vi "readFromXML.vi"(8 "error in (no error)":errorcluster, 10 "XML in":string, 11 "Guide in":refnum<class "Guide.lvclass">) -> (0 "error out":errorcluster, 3 "Guide out":refnum<class "Guide.lvclass">)   [LabVIEW 2022 SP3, in "TCSDataDefinitions.lvlib" / "TCSCommand.lvlib" / "GuiderCommands.lvlib" / "Guide.lvclass"]
uses:
  Guide.lvclass
  Enumerations/GuideStateTypes.ctl
  Guide.lvclass/Guide.ctl
  GuiderCommands.lvclass
  <userlib>/Common/XML/XMLParser/XMLParser.lvclass
  TCSCommand.lvlib
panel:
  out "guideStateTypes":T1
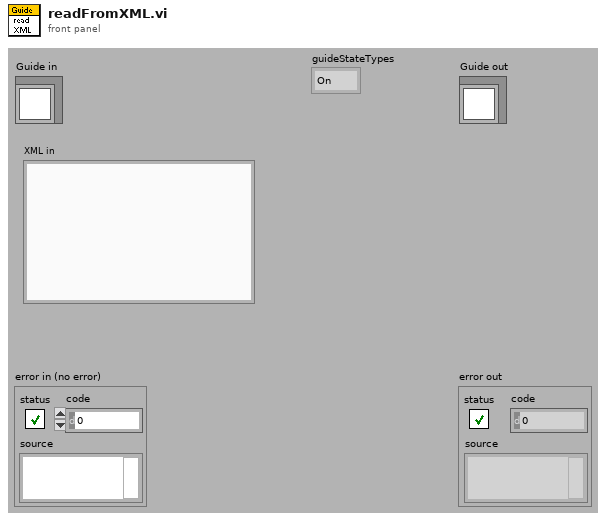
[diagram p1: front panel]
types:
  T1 = typedef "TCSDataDefinitions.lvlib/TCSCommand.lvlib/GuideStateTypes.ctl" = enum16{"On", "Off"}
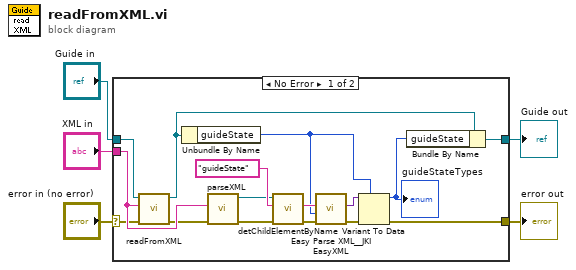
[diagram p0: block diagram]
diagram:
  n1 = case shown="No Error" "error in (no error)" {
    selector: "error in (no error)" -> [w15 w23]
    tunnel: [w9 w23] -> w4
    tunnel: [w19 w22] -> w2
    tunnel: "Guide in" -> [w18 w22]
    tunnel: "XML in" -> [w16 _]
    frame No Error {
      n2 = call-parent "readFromXML.vi"("error in (no error)"=w15, "XMLin"=w16, "GuiderCommands in"=w18) -> ("error out"=w14:errorcluster, "GuiderCommands out"=w17:refnum<class "Guide.lvclass">)  [unwired: 7 out]
      n3 = Unbundle By Name(w17) -> ("guideState"=w7:T1)
      n4 = call <userlib>:"parseXML.vi"("error in (no error)"=w14, "XMLString in"=w16) -> ("error out"=w20:errorcluster, "Element out"=w6:refnum<class "XMLParser.lvclass">)  [unwired: 8 in]
      n5 = call <userlib>:"detChildElementByName.vi"("error in (no error)"=w20, "childName"="guideState" ("ChildName"), "Element in"=w6) -> ("error out"=w10:errorcluster, "childXML"=w11:string)  [unwired: 5 in, 2 out]
      n6 = call <vilib>:"Easy Parse XML__JKI EasyXML.vi"("error in (no error)"=w10, "LabVIEW Data (Type)"=w7, "XML String"=w11) -> ("error out"=w13:errorcluster, "LabVIEW Data"=w12:variant)  [unwired: 7 in]
      n7 = Variant To Data(error in=w13, type=w7, Variant=w12) -> (data=w8:T1, error out=w9:errorcluster)
      "guideStateTypes" <- w8
      n8 = Bundle By Name(cluster=w17, "guideState"=w8) -> (w19:refnum<class "Guide.lvclass">)
    }
    frame Error {
    }
  }
  "error out" <- w4
  "Guide out" <- w2
